vi "Athermalize-focus.vi"(2 "Coefficient Thermique":dbl=2.75, 3 "temperature actuelle":dbl, 4 "Foyer à 0°":dbl) -> (0 "Foyer suggérer":i32)   [LabVIEW 2019]
panel:
  # "[ADU/°K]"
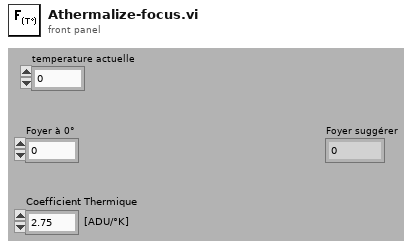
[diagram p1: front panel]
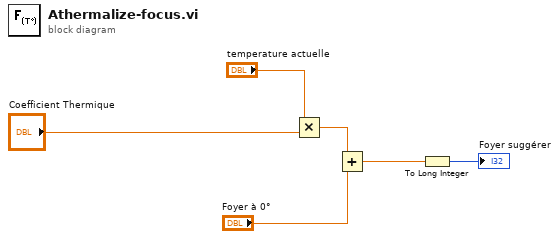
[diagram p0: block diagram]
diagram:
  n1 = Multiply(x="temperature actuelle", y="Coefficient Thermique") -> (x*y=w5:dbl)
  n2 = Add(x=w5, y="Foyer à 0°") -> (x+y=w4:dbl)
  n3 = To Long Integer(number=w4) -> (32bit integer=→"Foyer suggérer":i32)
